vi "MQTT_Disconnect.vi"(8 "error in (no error)":errorcluster, 11 "connection ID":refnum<k5>) -> (0 "error out":errorcluster)   [LabVIEW 2025, in "DAQIO MQTT.lvlib"]
doc: "Disconnects from an MQTT broker server.\n\n© 2015 - daq.io, LLC - Peter Adelhardt"
uses:
  DAQIO MQTT.lvlib
  Controls/MessageType.ctl
  Controls/Retain_Flag.ctl
  Controls/QoS.ctl
  Controls/DUP_Flag.ctl
  Controls/Conn_FGV_Cmds.ctl
  Controls/Conn_Stat_FGV_Cmds.ctl
  Controls/Connection_Return_Codes.ctl
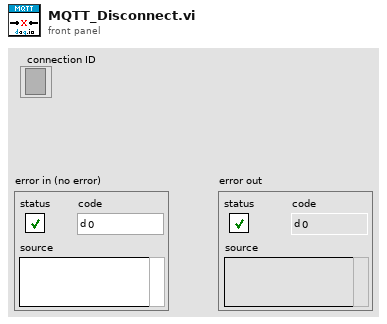
[diagram p1: front panel]
types:
  T1 = typedef "DAQIO MQTT.lvlib/Connection_Return_Codes.ctl" = enum16{"Connection accepted", "Connection refused: unacceptable protocol version", "Connection refused: identifier rejected", "Connection refused: Server unavailable", "Connection refused: bad user name or password", "Connection refused: not authorized"}
  T2 = typedef "DAQIO MQTT.lvlib/Conn_Stat_FGV_Cmds.ctl" = enum16{"Get", "Set"}
  T3 = typedef "DAQIO MQTT.lvlib/Conn_FGV_Cmds.ctl" = enum16{"Get", "Set", "Delete"}
  T4 = typedef "DAQIO MQTT.lvlib/DUP_Flag.ctl" = bool
  T5 = typedef "DAQIO MQTT.lvlib/QoS.ctl" = enum8{"At most once", "At least once", "Exactly once", "Reserved"}
  T6 = typedef "DAQIO MQTT.lvlib/Retain_Flag.ctl" = bool
  T7 = typedef "DAQIO MQTT.lvlib/MessageType.ctl" = enum32{"Reserved", "CONNECT", "CONNACK", "PUBLISH", "PUBACK", "PUBREC", "PUBREL", "PUBCOMP", "SUBSCRIBE", "SUBACK", "UNSUBSCRIBE", "UNSUBACK", "PINGREQ", "PINGRESP", "DISCONNECT", "Reserved2"}
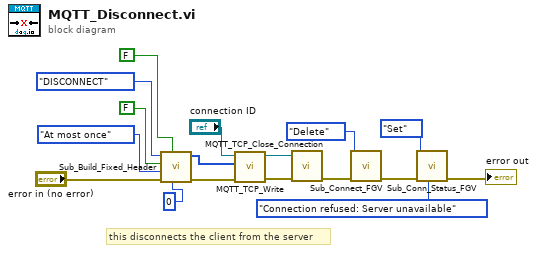
[diagram p0: block diagram]
diagram:
  # "this disconnects the client from the server"
  n1 = call "Sub_Build_Fixed_Header.vi"("Remaining Length"=u32 0, "Retain"=T6 FALSE, "error in (no error)"="error in (no error)", "QoS"=QoS."At most once", "DUP"=T4 FALSE, "MessageType"=MessageType."DISCONNECT") -> ("error out"=w11:errorcluster, "Fixed Header"=w10:u8[])  [unwired: 4 in]
  n2 = call "MQTT_TCP_Write.vi"("error in (no error)"=w11, "data in"=w10, "connection ID"="connection ID") -> ("error out"=w7:errorcluster, "connection ID out"=w8:refnum<k5>)  [unwired: 6 in, 1 out]
  n3 = call "MQTT_TCP_Close_Connection.vi"("error in (no error)"=w7, "connection ID"=w8) -> ("error out"=w6:errorcluster)  [unwired: 8 in, 1 out]
  n4 = call "Sub_Connect_FGV.vi"("error in"=w6, "Command"=Conn_FGV_Cmds."Delete") -> ("error out"=w4:errorcluster)  [unwired: 8 in, 1 out]
  n5 = call "Sub_Conn_Status_FGV.vi"("Connection Status in"=Connection_Return_Codes."Connection refused: Server unavailable", "error in"=w4, "Command"=Conn_Stat_FGV_Cmds."Set") -> ("error out"=→"error out":errorcluster)  [unwired: 7 in, 1 out]
